vi "Validate Serial Number.vi"(10 "Bypass Validation":bool, 11 "Serial Number":string) -> (2 "Valid SrNo?":bool, 3 "Reason":string)   [LabVIEW 2021, in "Sequence Engine.lvlib"]
uses:
  Sequence Engine.lvlib
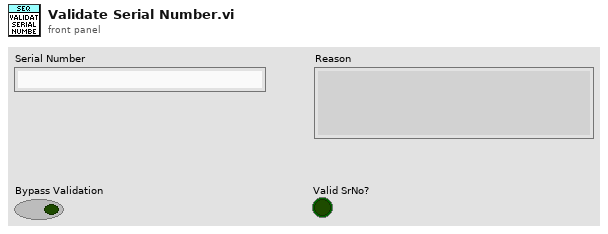
[diagram p1: front panel]
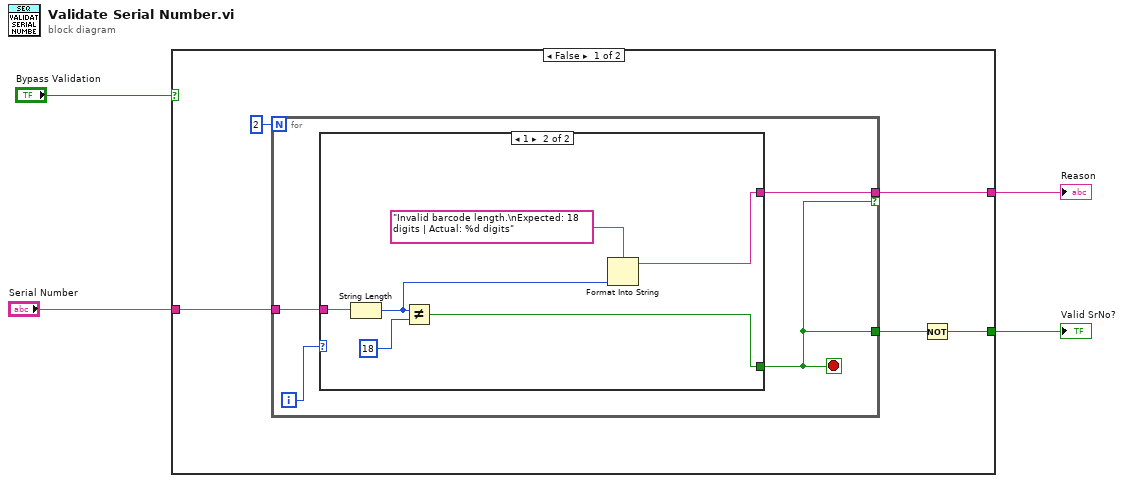
[diagram p0: block diagram]
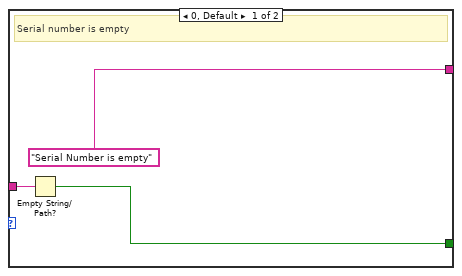
[diagram p2: hidden frame]
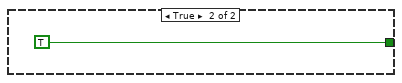
[diagram p3: hidden frame]
diagram:
  n1 = case shown="False" "Bypass Validation" {
    tunnel: [w9 _] -> w4
    tunnel: "Serial Number" -> [w7 _]
    tunnel: [w5 TRUE] -> w2
    frame False {
      n2 = for {
        N: 2 -> [_]
        tunnel: w7 -> [w13]
        tunnel: [w11] -> w9 if=w10
        tunnel: [w10] -> w6
        i -> [w12]
        stop <- w10 stop-if-true
        n3 = case shown="1" w12 {
          tunnel: w13 -> [w16 w22]
          tunnel: [w15 w20] -> w10
          tunnel: ["Serial Number is empty" ("Reason") w17] -> w11
          frame 0, Default {
            # "Serial number is empty"
            n4 = Empty String/Path?(string/path=w16) -> (empty?=w15:bool)
          }
          frame 1 {
            n5 = String Length(string=w22) -> (length=w18:i32)
            n6 = Not Equal?(x=w18, y=18) -> (x != y?=w20:bool)
            n7 = Format Into String(format string="Invalid barcode length.\nExpected: 18 digits | Actual: %d digits" ("Reason"), w18) -> (resulting string=w17:string)  [unwired: 2 in, 1 out]
          }
        }
      }
      n8 = Not(x=w6) -> (.not. x?=w5:bool)
    }
    frame True {
    }
  }
  "Reason" <- w4
  "Valid SrNo?" <- w2
